vi "Exercise4.2-Pre-Lab2-2.vi"() -> ()   [LabVIEW 2013]
uses:
  <vilib>/express/express analysis/Spectral/Block/exnSpectralBlock spectral measurements RMS poly.vi
  <vilib>/express/express analysis/Spectral/Block/exnSpectralBlock spectral measurements RMS DDT.vi
  <vilib>/express/express analysis/Spectral/XNode/ExpressSpectralMeasurementsBlockNode.xnode
panel:
  out "Spectrum":dynamicdata(graph)=[{"t0"=timestamp(0 s since 1904-01-01), "dt"=1.0040160642570282, "Y"=array[498 elements], "attributes"=variant("NI_ChannelName"=variant(string "Sine (FFT - (RMS))"), "NI_ExpIsRelativeTime"=variant(bool TRUE), "NI_ExpStartTimeStamp"=variant(timestamp timestamp(3695350991.724483 s since 1904-01-01)), "NI_ExpTimeStamp"=variant(timestamp timestamp(3695350991.724483 s since 1904-01-01)), "NI_ExpXDimension"=variant(string "f"), "NI_OriginalChannelName"=variant(string "Sine"))}, {"t0"=timestamp(0 s since 1904-01-01), "dt"=1.0, "Y"=array[500 elements], "attributes"=variant("NI_ChannelName"=variant(string "Sine (FFT - (RMS))"), "NI_ExpIsRelativeTime"=variant(bool TRUE), "NI_ExpStartTimeStamp"=variant(timestamp timestamp(3695350991.78835 s since 1904-01-01)), "NI_ExpTimeStamp"=variant(timestamp timestamp(3695350991.78835 s since 1904-01-01)), "NI_ExpXDimension"=variant(string "f"), "NI_OriginalChannelName"=variant(string "Sine"))}, {"t0"=timestamp(0 s since 1904-01-01), "dt"=1.0040160642570282, "Y"=array[498 elements], "attributes"=variant("NI_ChannelName"=variant(string "Sine (FFT - (RMS))"), "NI_ExpIsRelativeTime"=variant(bool TRUE), "NI_ExpStartTimeStamp"=variant(timestamp timestamp(3695350991.724483 s since 1904-01-01)), "NI_ExpTimeStamp"=variant(timestamp timestamp(3695350991.724483 s since 1904-01-01)), "NI_ExpXDimension"=variant(string "f"), "NI_OriginalChannelName"=variant(string "Sine"))}]
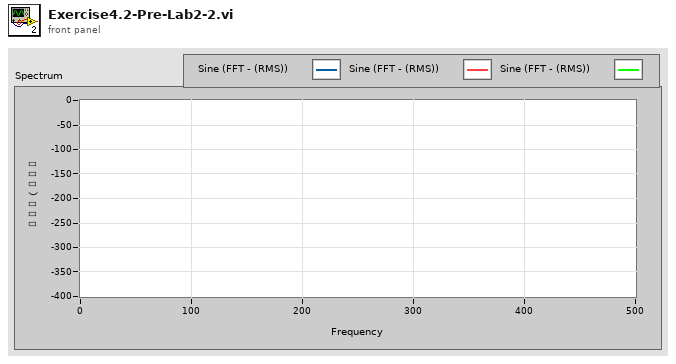
[diagram p1: front panel]
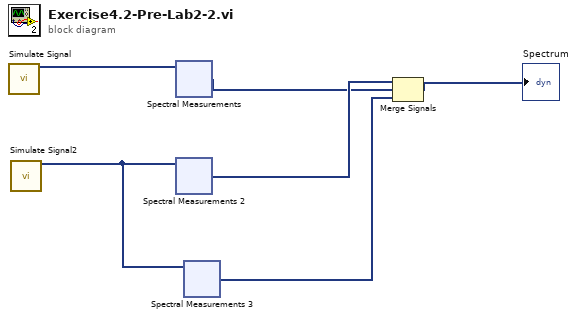
[diagram p0: block diagram]
diagram:
  n1 = call "Simulate Signal"() -> ("Sine"=w6:dynamicdata)  [unwired: 14 in, 1 out]
  n2 = call "Simulate Signal2"() -> ("Sine"=w2:dynamicdata)  [unwired: 14 in, 1 out]
  n3 = xnode "Spectral Measurements"("Signals"=w6) -> ("FFT - (RMS)"=w3:dynamicdata)  [unwired: 1 in, 2 out]
  n4 = xnode "Spectral Measurements 2"("Signals"=w2) -> ("FFT - (RMS)"=w4:dynamicdata)  [unwired: 1 in, 2 out]
  n5 = xnode "Spectral Measurements 3"("Signals"=w2) -> ("FFT - (RMS)"=w1:dynamicdata)  [unwired: 1 in, 2 out]
  n6 = Merge Signals(w4, w3, w1) -> (→"Spectrum":dynamicdata)
